vi "Step.vi"(8 "error in":errorcluster, 11 "VISA resource name":refnum<visa-resource-name>) -> (0 "error out":errorcluster, 3 "VISA resource name out":refnum<visa-resource-name>)   [LabVIEW 2016, in "Andeen-Hagerling 2550.lvlib"]
doc: "This VI causes the bridge to execute a single measurement and iterate through coupled parameter values when paramater scanning is enabled."
uses:
  Andeen-Hagerling 2550.lvlib
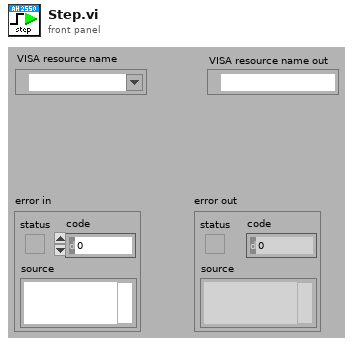
[diagram p1: front panel]
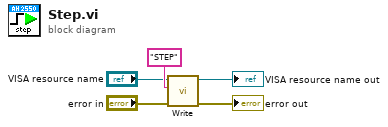
[diagram p0: block diagram]
diagram:
  n1 = call "Write.vi"("error in"="error in", "command"="STEP", "VISA resource name"="VISA resource name") -> ("error out"=→"error out":errorcluster, "VISA resource name out"=→"VISA resource name out":refnum<visa-resource-name>)  [unwired: 7 in]
